vi "1 port_Capacitance Parameters.vi"(0 "Port Measurements":T1, 2 "Specific Voltages":dbl[](array[numeric])=[32.0, 36.0], 5 "Selected Exp Settings":T2={"Floor_Sweep_Stop_V"=36.0, "Resistance Threshold"=1.0, "Floor_Sweep_Start_V"=36.0, "Floor_Sweep_Step_V"=1.0, "Roof_Sweep_Stop_V"=36.0, "Roof_Sweep_Start_V"=36.0, "Roof_Sweep_Step_V"=1.0, "Experiment Name"="", "Meas_Type"=[0, 2, 4]}, 11 "Error In":errorcluster) -> (4 "Port Capacitance Parametic Calculations":T4, 15 "Error Out":errorcluster)   [LabVIEW 2013]
uses:
  Controls/Port Measurements.ctl
  Controls/Port Capacitance Parametric Calculations.ctl
  Controls/Individual User Inputs_MultiTest.ctl
  Controls/Test Selection.ctl
panel:
  in  "Tab Control":enum32{"Inputs", "Outputs"}(tab)
  # "Calculation Settings"
  # "Test Settings"
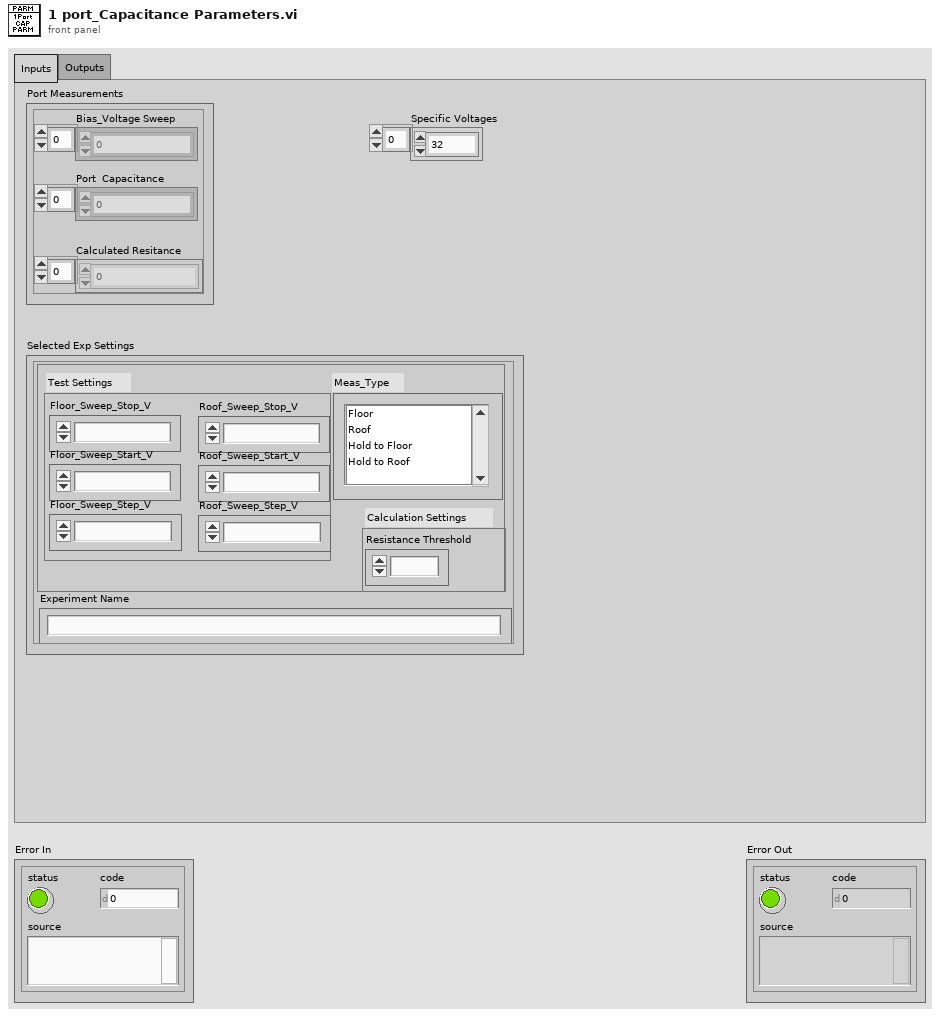
[diagram p1: front panel]
types:
  T1 = typedef "Port Measurements.ctl" = cluster{"Bias_Voltage Sweep":dbl[], "Port  Capacitance":dbl[], "Calculated Resitance":dbl[]}
  T2 = typedef "Individual User Inputs_MultiTest.ctl" = cluster{"Floor_Sweep_Stop_V":dbl, "Resistance Threshold":dbl, "Floor_Sweep_Start_V":dbl, "Floor_Sweep_Step_V":dbl, "Roof_Sweep_Stop_V":dbl, "Roof_Sweep_Start_V":dbl, "Roof_Sweep_Step_V":dbl, "Experiment Name":string, "Meas_Type":T3}
  T3 = typedef "Test Selection.ctl" = i32[]
  T4 = typedef "Port Capacitance Parametric Calculations.ctl" = cluster{"C_free":dbl, "C_vmax":dbl, "C_first":dbl, "C_last":dbl, "C_end":dbl, "Meas@Specific Voltages":dbl[]}
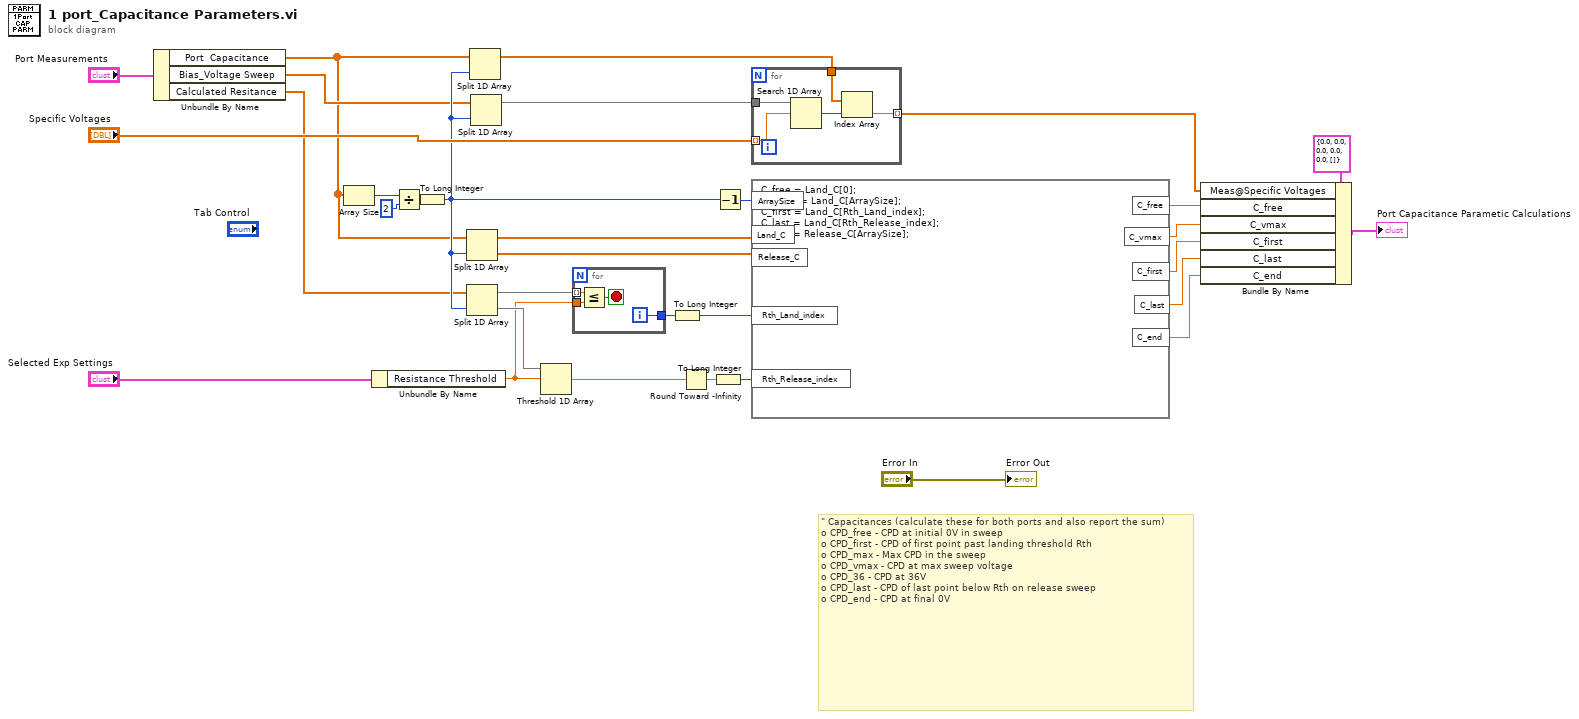
[diagram p0: block diagram]
diagram:
  # "\"\tCapacitances (calculate these for both ports and also report the sum)\no\tCPD_free - CPD at initial 0V in sweep\no\tCPD_first - CPD of first point past landing threshold Rth \no\tCPD_max - Max CPD in the sweep\no\tCPD_vmax - CPD at max sweep voltage\no\tCPD_36 - CPD at 36V\no\tCPD_last - CPD of last point below Rth on release sweep\no\tCPD_end - CPD at final 0V"
  n1 = Unbundle By Name("Port Measurements") -> ("Port  Capacitance"=w11:dbl[], "Bias_Voltage Sweep"=w12:dbl[], "Calculated Resitance"=w10:dbl[])
  n2 = Array Size(array=w11) -> (size(s)=w32:i32)
  n3 = Unbundle By Name("Selected Exp Settings") -> ("Resistance Threshold"=w15:dbl)
  n4 = Divide(x=w32, y=2) -> (x/y=w30:dbl)
  n5 = To Long Integer(number=w30) -> (32bit integer=w21:i32)
  n6 = Split 1D Array(array=w11, index=w21) -> (first subarray=w23:dbl[], second subarray=w24:dbl[])
  n7 = Split 1D Array(array=w10, index=w21) -> (first subarray=w16:dbl[], second subarray=w28:dbl[])
  n8 = Split 1D Array(array=w11, index=w21) -> (first subarray=w19:dbl[])  [unwired: 1 out]
  n9 = Split 1D Array(array=w12, index=w21) -> (first subarray=w18:dbl[])  [unwired: 1 out]
  n10 = Threshold 1D Array(2:w15, 3:w28) -> (0:w27:dbl)  [unwired: 1 in]
  n11 = for {
    tunnel: [w36] -> w14
    tunnel: w16 -> [w34] mode=indexing
    tunnel: w15 -> [w33]
    i -> [w36]
    stop <- w35 stop-if-true
    n12 = Less Or Equal?(x=w34, y=w33) -> (x <= y?=w35:bool)
  }
  n13 = To Long Integer(number=w14) -> (32bit integer=w29:i32)
  n14 = Round Toward -Infinity(1:w27) -> (0:w26:dbl)
  n15 = To Long Integer(number=w26) -> (32bit integer=w25:i32)
  n16 = Decrement(x=w21) -> (x-1=w20:i32)
  n17 = for {
    tunnel: "Specific Voltages" -> [w41] mode=indexing
    tunnel: w18 -> [w40]
    tunnel: w19 -> [w38]
    tunnel: [w37] -> w8 mode=indexing
    n18 = Search 1D Array(1D array=w40, element=w41) -> (index of element=w39:i32)  [unwired: 1 in]
    n19 = Index Array(array=w38, index=w39) -> (element=w37:dbl)
  }
  n20 = formula code="C_free = Land_C[0];\nC_vmax = Land_C[ArraySize];\nC_first = Land_C[Rth_Land_index];\nC_last = Land_C[Rth_Release_index];\nC_end = Release_C[ArraySize];"("Land_C"=w23, "ArraySize"=w20, "Rth_Land_index"=w29, "Rth_Release_index"=w25, "Release_C"=w24) -> ("C_free"=w7:dbl, "C_vmax"=w6:dbl, "C_first"=w5:dbl, "C_last"=w4:dbl, "C_end"=w3:dbl)
  n21 = Bundle By Name(cluster=T4 {"C_free"=0.0, "C_vmax"=0.0, "C_first"=0.0, "C_last"=0.0, "C_end"=0.0, "Meas@Specific Voltages"=[]} ("Port Parametic Calculations 2"), "Meas@Specific Voltages"=w8, "C_free"=w7, "C_vmax"=w6, "C_first"=w5, "C_last"=w4, "C_end"=w3) -> (→"Port Capacitance Parametic Calculations":T4)
  "Error Out" <- "Error In"
